vi "AlliGator Bin Simple Image.vi"(8 "error in (no error)":errorcluster, 10 "Image Binning Options":T1={"Use Image Binning"=FALSE, "X Bin"=1, "Y Bin"=1} {"Y Bin" min=1; "X Bin" min=1}, 11 "Refnum in":T2) -> (0 "error out":errorcluster, 3 "Refnum out":T2)   [LabVIEW 2021, in "AlliGator Source Image.lvlib"]
doc: "Bins an image according to the Settings:Source Image:<B>Image Binning Options</B>."
uses:
  AlliGator Source Image.lvlib
  <vilib>/vision/Image Controls.llb/IMAQ Image.ctl
  AlliGator Image Binning Options.ctl
  8795834c-7319-4b1e-863e-cb668b9e48b5.vi
  a6de7b5c-2a9e-481d-8f0f-7c805359ca0d.vi
  1f3143f1-d618-433b-a838-af458d24a5e4.vi
  6ac41207-3708-4752-af93-ce9f4deff1c2.vi
  Time/High Resolution Timing.vi
panel:
  # "see the AlliGator License on the block diagram (Ctrl+E or Window:Show Block Diagram)"
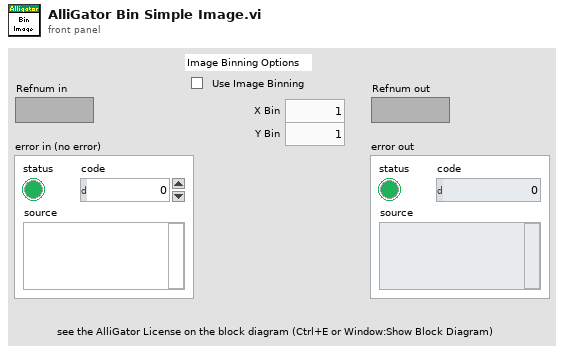
[diagram p1: front panel]
types:
  T1 = typedef "AlliGator Source Image.lvlib/AlliGator Image Binning Options.ctl" = cluster{"Use Image Binning":bool, "X Bin":i32, "Y Bin":i32}
  T2 = typedef "IMAQ Image.ctl" = refnum<image>
  T3 = typedef "Image Type" = u32
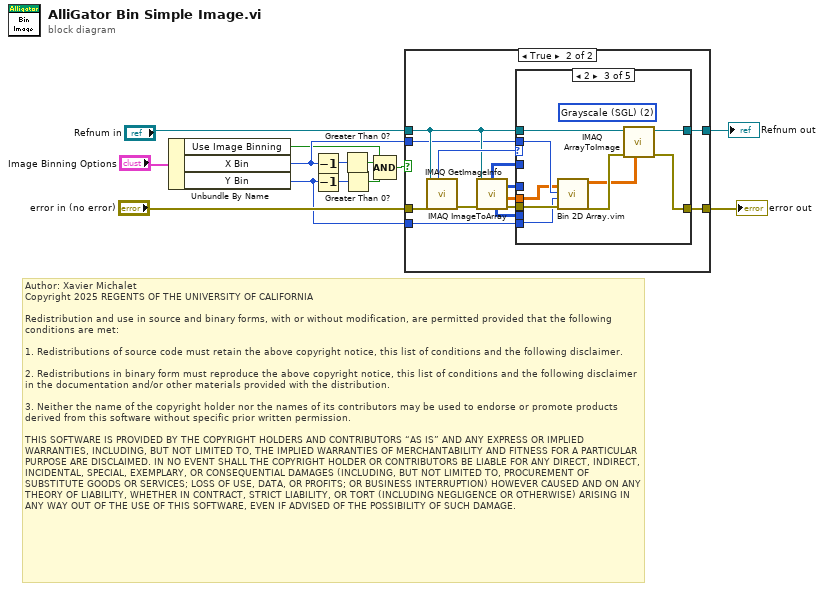
[diagram p0: block diagram]
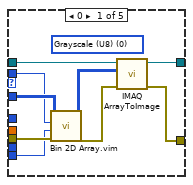
[diagram p3: hidden frame]
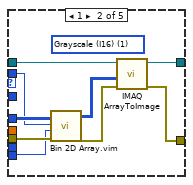
[diagram p4: hidden frame]
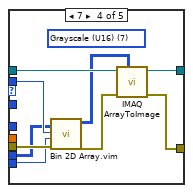
[diagram p5: hidden frame]
diagram:
  # "Author: Xavier Michalet\nCopyright 2025 REGENTS OF THE UNIVERSITY OF CALIFORNIA\n\nRedistribution and use in source and binary forms, with or without modification, are permitted provided that the following conditions are met:\n\n1. Redistributions of source code must retain the above copyright notice, this list of conditions and the following disclaimer.\n\n2. Redistributions in binary form must reproduce the above copyright notice, this list of conditions and the following disclaimer in the documentation and/or other materials provided with the distribution.\n\n3. Neither the name of the copyright holder nor the names of its contributors may be used to endorse or promote products derived from this software without specific prior written permission.\n\nTHIS SOFTWARE IS PROVIDED BY THE COPYRIGHT HOLDERS AND CONTRIBUTORS “AS IS” AND ANY EXPRESS OR IMPLIED WARRANTIES, INCLUDING, BUT NOT LIMITED TO, THE IMPLIED WARRANTIES OF MERCHANTABILITY AND FITNESS FOR A PARTICULAR PURPOSE ARE DISCLAIMED. IN NO EVENT SHALL THE COPYRIGHT HOLDER OR CONTRIBUTORS BE LIABLE FOR ANY DIRECT, INDIRECT, INCIDENTAL, SPECIAL, EXEMPLARY, OR CONSEQUENTIAL DAMAGES (INCLUDING, BUT NOT LIMITED TO, PROCUREMENT OF SUBSTITUTE GOODS OR SERVICES; LOSS OF USE, DATA, OR PROFITS; OR BUSINESS INTERRUPTION) HOWEVER CAUSED AND ON ANY THEORY OF LIABILITY, WHETHER IN CONTRACT, STRICT LIABILITY, OR TORT (INCLUDING NEGLIGENCE OR OTHERWISE) ARISING IN ANY WAY OUT OF THE USE OF THIS SOFTWARE, EVEN IF ADVISED OF THE POSSIBILITY OF SUCH DAMAGE."
  n1 = Unbundle By Name("Image Binning Options") -> ("Use Image Binning"=w1:bool, "X Bin"=w3:i32, "Y Bin"=w2:i32)
  n2 = Decrement(x=w3) -> (x-1=w8:i32)
  n3 = Decrement(x=w2) -> (x-1=w7:i32)
  n4 = Greater Than 0?(x=w8) -> (x > 0?=w6:bool)
  n5 = Greater Than 0?(x=w7) -> (x > 0?=w5:bool)
  n6 = Compound Arithmetic op=AND(w1, w6, w5) -> (w4:bool)
  n7 = case shown="True" w4 {
    tunnel: [w14 w25] -> w13
    tunnel: "error in (no error)" -> [w14 w28]
    tunnel: [w15 w21] -> w11
    tunnel: "Refnum in" -> [w15 w22]
    tunnel: w3 -> [_ w19]
    tunnel: w2 -> [_ w18]
    frame False {
    }
    frame True {
      n8 = call "IMAQ GetImageInfo"("error in (no error)"=w28, "Image"=w22) -> ("error out"=w27:errorcluster, "Image Type"=w24:T3)  [unwired: 2 in, 6 out]
      n9 = call "IMAQ ImageToArray"("error in (no error)"=w27, "Image"=w22) -> ("Image Pixels (U16)"=w16:u16[][], "Image Pixels (Float)"=w17:sgl[][], "error out"=w26:errorcluster, "Image Pixels (U8)"=w23:u8[][], "Image Pixels (I16)"=w20:i16[][])  [unwired: 2 in]
      n10 = case shown="2" w24 {
        tunnel: w26 -> [w37 w46 w55 w64 w65]
        tunnel: [w31 w42 w51 w60 w65] -> w25
        tunnel: w23 -> [w36 _ _ _ _]
        tunnel: w22 -> [w35 w45 w54 w63 w66]
        tunnel: [w33 w44 w53 w62 w66] -> w21
        tunnel: w20 -> [_ w41 _ _ _]
        tunnel: w19 -> [w30 w39 w50 w59 _]
        tunnel: w18 -> [w29 w38 w49 w58 _]
        tunnel: w17 -> [_ _ w48 _ _]
        tunnel: w16 -> [_ _ _ w57 _]
        frame 0 {
          (unwired) T3 0 items=["Grayscale (U8)", "Grayscale (I16)", "Grayscale (SGL)", "Complex (CSG)", "RGB (U32)", "HSL (U32)", "RGB (U64)", "Grayscale (U16)"] ("Image Type")
          n11 = call "Bin 2D Array.vim"("Error In"=w37, "Y Bin (1)"=w29, "X Bin (1)"=w30, "Array"=w36) -> ("Error Out"=w32:errorcluster, "Binned Array"=w34:u8[][])  [unwired: 2 in, 4 out]
          n12 = call "IMAQ ArrayToImage"("error in (no error)"=w32, "Image Pixels (U8)"=w34, "Image"=w35) -> ("error out"=w31:errorcluster, "Image Out"=w33:T2)  [unwired: 7 in]
        }
        frame 1 {
          (unwired) T3 1 items=["Grayscale (U8)", "Grayscale (I16)", "Grayscale (SGL)", "Complex (CSG)", "RGB (U32)", "HSL (U32)", "RGB (U64)", "Grayscale (U16)"] ("Image Type")
          n13 = call "Bin 2D Array.vim"("Error In"=w46, "Y Bin (1)"=w38, "X Bin (1)"=w39, "Array"=w41) -> ("Error Out"=w43:errorcluster, "Binned Array"=w40:i16[][])  [unwired: 2 in, 4 out]
          n14 = call "IMAQ ArrayToImage"("error in (no error)"=w43, "Image Pixels (I16)"=w40, "Image"=w45) -> ("error out"=w42:errorcluster, "Image Out"=w44:T2)  [unwired: 7 in]
        }
        frame 2 {
          (unwired) T3 2 items=["Grayscale (U8)", "Grayscale (I16)", "Grayscale (SGL)", "Complex (CSG)", "RGB (U32)", "HSL (U32)", "RGB (U64)", "Grayscale (U16)"] ("Image Type")
          n15 = call "Bin 2D Array.vim"("Error In"=w55, "Y Bin (1)"=w49, "X Bin (1)"=w50, "Array"=w48) -> ("Error Out"=w52:errorcluster, "Binned Array"=w47:sgl[][])  [unwired: 2 in, 4 out]
          n16 = call "IMAQ ArrayToImage"("Image Pixels (Float)"=w47, "error in (no error)"=w52, "Image"=w54) -> ("error out"=w51:errorcluster, "Image Out"=w53:T2)  [unwired: 7 in]
        }
        frame 7 {
          (unwired) T3 7 items=["Grayscale (U8)", "Grayscale (I16)", "Grayscale (SGL)", "Complex (CSG)", "RGB (U32)", "HSL (U32)", "RGB (U64)", "Grayscale (U16)"] ("Image Type")
          n17 = call "Bin 2D Array.vim"("Error In"=w64, "Y Bin (1)"=w58, "X Bin (1)"=w59, "Array"=w57) -> ("Error Out"=w61:errorcluster, "Binned Array"=w56:u16[][])  [unwired: 2 in, 4 out]
          n18 = call "IMAQ ArrayToImage"("Image Pixels (U16)"=w56, "error in (no error)"=w61, "Image"=w63) -> ("error out"=w60:errorcluster, "Image Out"=w62:T2)  [unwired: 7 in]
        }
        frame 3, Default {
        }
      }
    }
  }
  "error out" <- w13
  "Refnum out" <- w11
